vi "Main.vi"() -> ()   [LabVIEW 2015]
uses:
  <vilib>/NXT/Block Support/NXT_InputPort.ctl
  <vilib>/NXT/Subs/ColorSensorColors.ctl
  <vilib>/NXT/Block Support/NXT_OutputPort.ctl
  <vilib>/NXT/Dual Mode Library/Sensors/EV3_Color_Color.vi
  <vilib>/NXT/Dual Mode Library/Sensors/Touch_Released.vi
  <vilib>/NXT/Dual Mode Library/Sound/Tone.vi
  <vilib>/NXT/Dual Mode Library/Sensors/Read_NewTemp.vi
  <vilib>/NXT/NXTIO Xnodes/NXTIONodeSubVIs/NXTStopMotors.vi
  <vilib>/NXT/NXTIO Xnodes/NXTIONodeSubVIs/NXTMoveMotors.vi
  <vilib>/NXT/Dual Mode Library/Sensors/EV3_Color_Ambient.vi
  <vilib>/NXT/NXTIO Xnodes/AddressXNode/NXTIOAddress.xnode
  <vilib>/NXT/Subs/LVHSConnector.ctl
  <vilib>/NXT/NXTIO Xnodes/NXTIOXNode/NXTIO.xnode
  <vilib>/NXT/LegoClasses/BrickReference/BrickReference.lvclass
panel:
  out "String":string
  in  "Knob 2":dbl(knob) scale=0.0..100.0
  out "Numeric Indicator":dbl
  in  "Knob":dbl(knob) scale=0.0..100.0
  # "Управление температурой"
  # "ТЕКУЩАЯ ТЕМПЕРАТУРА В BIObox"
  # "Т"
  # "Управление освещенностью"
  # "ГРАДУСОВ ПО ЦЕЛЬСИЮ"
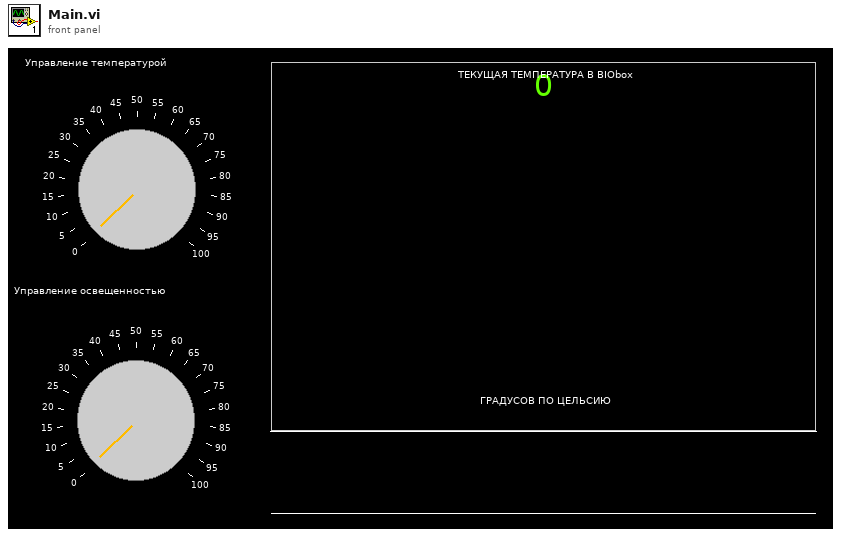
[diagram p1: front panel]
types:
  T1 = typedef "NXT_InputPort.ctl" = u32
  T2 = typedef "ColorSensorColors.ctl" = enum16{"No Color", "Black", "Blue", "Green", "Yellow", "Red", "White", "Brown"}
  T3 = typedef "NXT_OutputPort.ctl" = u8
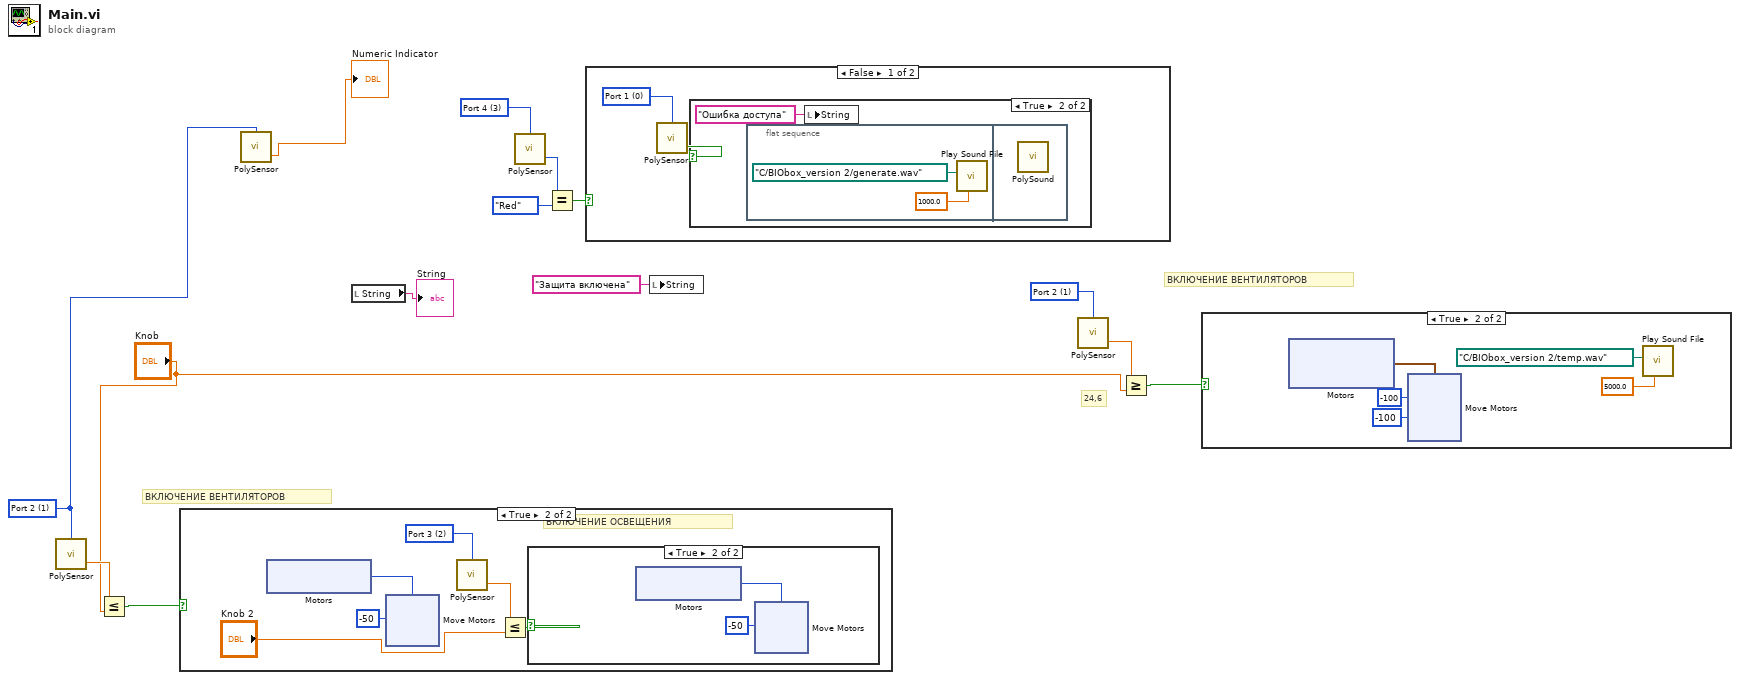
[diagram p0: block diagram]
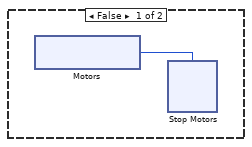
[diagram p2: hidden frame]
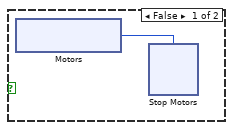
[diagram p3: hidden frame]
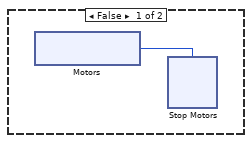
[diagram p4: hidden frame]
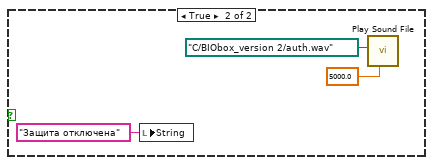
[diagram p6: hidden frame]
diagram:
  w4 = T1 1 items=["Port 1", "Port 2", "Port 3", "Port 4"] ("Port (Port 1)")
  w8 = T1 1 items=["Port 1", "Port 2", "Port 3", "Port 4"] ("Port (Port 1)")
  w14 = T1 3 items=["Port 1", "Port 2", "Port 3", "Port 4"] ("Port (Port 1)")
  # "24,6"
  # "ВКЛЮЧЕНИЕ ВЕНТИЛЯТОРОВ"
  # "ВКЛЮЧЕНИЕ ВЕНТИЛЯТОРОВ"
  n1 = call-poly <vilib>:"PolySensor.vi"("Port (Port 4)"=w4) -> ("Celsius"=w6:sgl)  [unwired: 2 in, 1 out]
  n2 = Less Or Equal?(x=w6, y="Knob") -> (x <= y?=w7:bool)
  n3 = case shown="True" w7 {
    frame False {
      n4 = xnode "Motors"() -> ("Motor"=w15:T3)
      n5 = xnode "Stop Motors"("Motors"=w15) -> ()  [unwired: 1 in, 1 out]
    }
    frame True {
      w25 = T1 2 items=["Port 1", "Port 2", "Port 3", "Port 4"] ("Port (Port 1)")
      # "ВКЛЮЧЕНИЕ ОСВЕЩЕНИЯ"
      n6 = xnode "Motors"() -> ("Motor"=w27:T3)
      n7 = xnode "Move Motors"("Power/Speed 1"=i8 -50, "Motors"=w27) -> ()  [unwired: 1 in, 1 out]
      n8 = call-poly <vilib>:"PolySensor.vi"("Port (Port 1)"=w25) -> ("Scaled Value"=w24:sgl)  [unwired: 2 in, 1 out]
      n9 = Less Or Equal?(x=w24, y="Knob 2") -> (x <= y?=w23:bool)
      n10 = case shown="True" w23 {
        frame False {
          n11 = xnode "Motors"() -> ("Motor"=w28:T3)
          n12 = xnode "Stop Motors"("Motors"=w28) -> ()  [unwired: 1 in, 1 out]
        }
        frame True {
          n13 = xnode "Motors"() -> ("Motor"=w35:T3)
          n14 = xnode "Move Motors"("Power/Speed 1"=i8 -50, "Motors"=w35) -> ()  [unwired: 1 in, 1 out]
        }
      }
    }
  }
  n15 = call-poly <vilib>:"PolySensor.vi"("Port (Port 4)"=w4) -> ("Celsius"=→"Numeric Indicator":sgl)  [unwired: 2 in, 1 out]
  n16 = local read "String"() -> (→"String":string)
  n17 = call-poly <vilib>:"PolySensor.vi"("Port (Port 1)"=w14) -> ("Detected Color"=w12:T2)  [unwired: 2 in, 1 out]
  n18 = Equal?(x=w12, y=ColorSensorColors."Red") -> (x = y?=w13:bool)
  n19 = case shown="False" w13 {
    frame False {
      w53 = T1 0 items=["Port 1", "Port 2", "Port 3", "Port 4"] ("Port (Port 1)")
      n20 = call-poly <vilib>:"PolySensor.vi"("Port (Port 1)"=w53) -> ("Yes / No"=w54:bool)  [unwired: 2 in, 1 out]
      n21 = case shown="True" w54 {
        frame False {
        }
        frame True {
          n22 = flat-sequence {
            frame #0 {
              n23 = call <vilib>:"Play Sound File.vi"("timeout (sec)"=1000.0, "path"=path "C:/BIObox_version 2/generate.wav") -> ()  [unwired: 8 in, 2 out]
            }
            frame #1 {
              n24 = call-poly <vilib>:"PolySound.vi"() -> ()  [unwired: 4 in, 1 out]
            }
          }
          n25 = local write "String"("Ошибка доступа" ("String")) -> ()
        }
      }
    }
    frame True {
      n26 = local write "String"("Защита отключена" ("String")) -> ()
      n27 = call <vilib>:"Play Sound File.vi"("timeout (sec)"=5000.0, "path"=path "C:/BIObox_version 2/auth.wav") -> ()  [unwired: 8 in, 2 out]
    }
  }
  n28 = local write "String"("Защита включена" ("String")) -> ()
  n29 = call-poly <vilib>:"PolySensor.vi"("Port (Port 4)"=w8) -> ("Celsius"=w9:sgl)  [unwired: 2 in, 1 out]
  n30 = Greater Or Equal?(x=w9, y="Knob") -> (x >= y?=w10:bool)
  n31 = case shown="True" w10 {
    frame False {
      n32 = xnode "Motors"() -> ("Motor"=w61:T3)
      n33 = xnode "Stop Motors"("Motors"=w61) -> ()  [unwired: 1 in, 1 out]
    }
    frame True {
      n34 = xnode "Motors"() -> ("Motor"=w72:cluster{"Port":T3, "Port":T3})
      n35 = xnode "Move Motors"("Power/Speed 2"=i8 -100, "Power/Speed 1"=i8 -100, "Motors"=w72) -> ()  [unwired: 1 in, 1 out]
      n36 = call <vilib>:"Play Sound File.vi"("timeout (sec)"=5000.0, "path"=path "C:/BIObox_version 2/temp.wav") -> ()  [unwired: 8 in, 2 out]
    }
  }
